vi "Close.vi"(8 "error in (no error)":errorcluster, 11 "MenuButton Event Handler in":refnum<class "MenuButton Event Handler.lvclass">) -> (0 "error out":errorcluster)   [LabVIEW 2017, in "MenuButtons.lvlib" / "MenuButton Event Handler.lvclass"]
uses:
  MenuButton Event Handler.lvclass
  MenuButton Event Handler.lvclass/MenuButton Event Handler.ctl
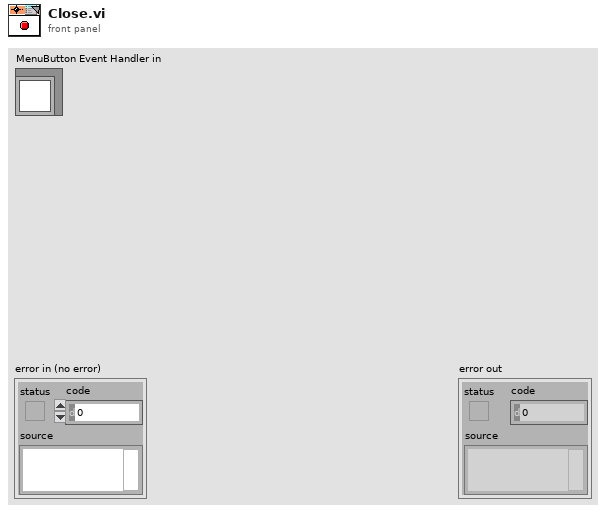
[diagram p1: front panel]
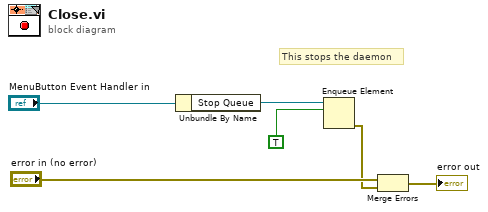
[diagram p0: block diagram]
diagram:
  # "This stops the daemon"
  n1 = Unbundle By Name("MenuButton Event Handler in") -> ("Stop Queue"=w4:refnum<queue>)
  n2 = Enqueue Element(queue=w4, element=TRUE) -> (error out=w1:errorcluster)  [unwired: 2 in, 2 out]
  n3 = Merge Errors("error in (no error)", w1) -> (→"error out":errorcluster)
